vi "SetDisplayState.vi"(8 "Error In":errorcluster, 10 "Enabled?":bool, 11 "Keithley 6485 In":refnum<visa-resource-name>) -> (0 "Error Out":errorcluster, 3 "Keithley 6485 Out":refnum<visa-resource-name>)   [LabVIEW 2012, in "Keithley-6485.lvlib"]
uses:
  Keithley-6485.lvlib
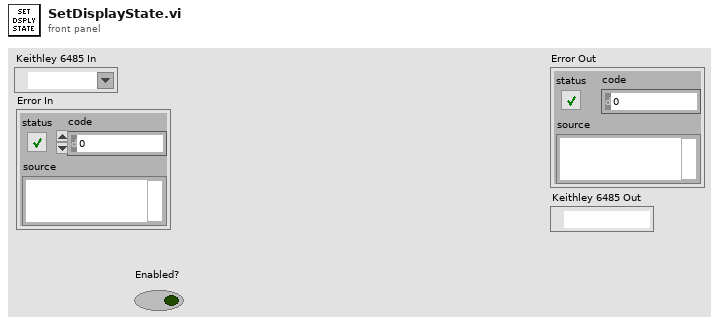
[diagram p1: front panel]
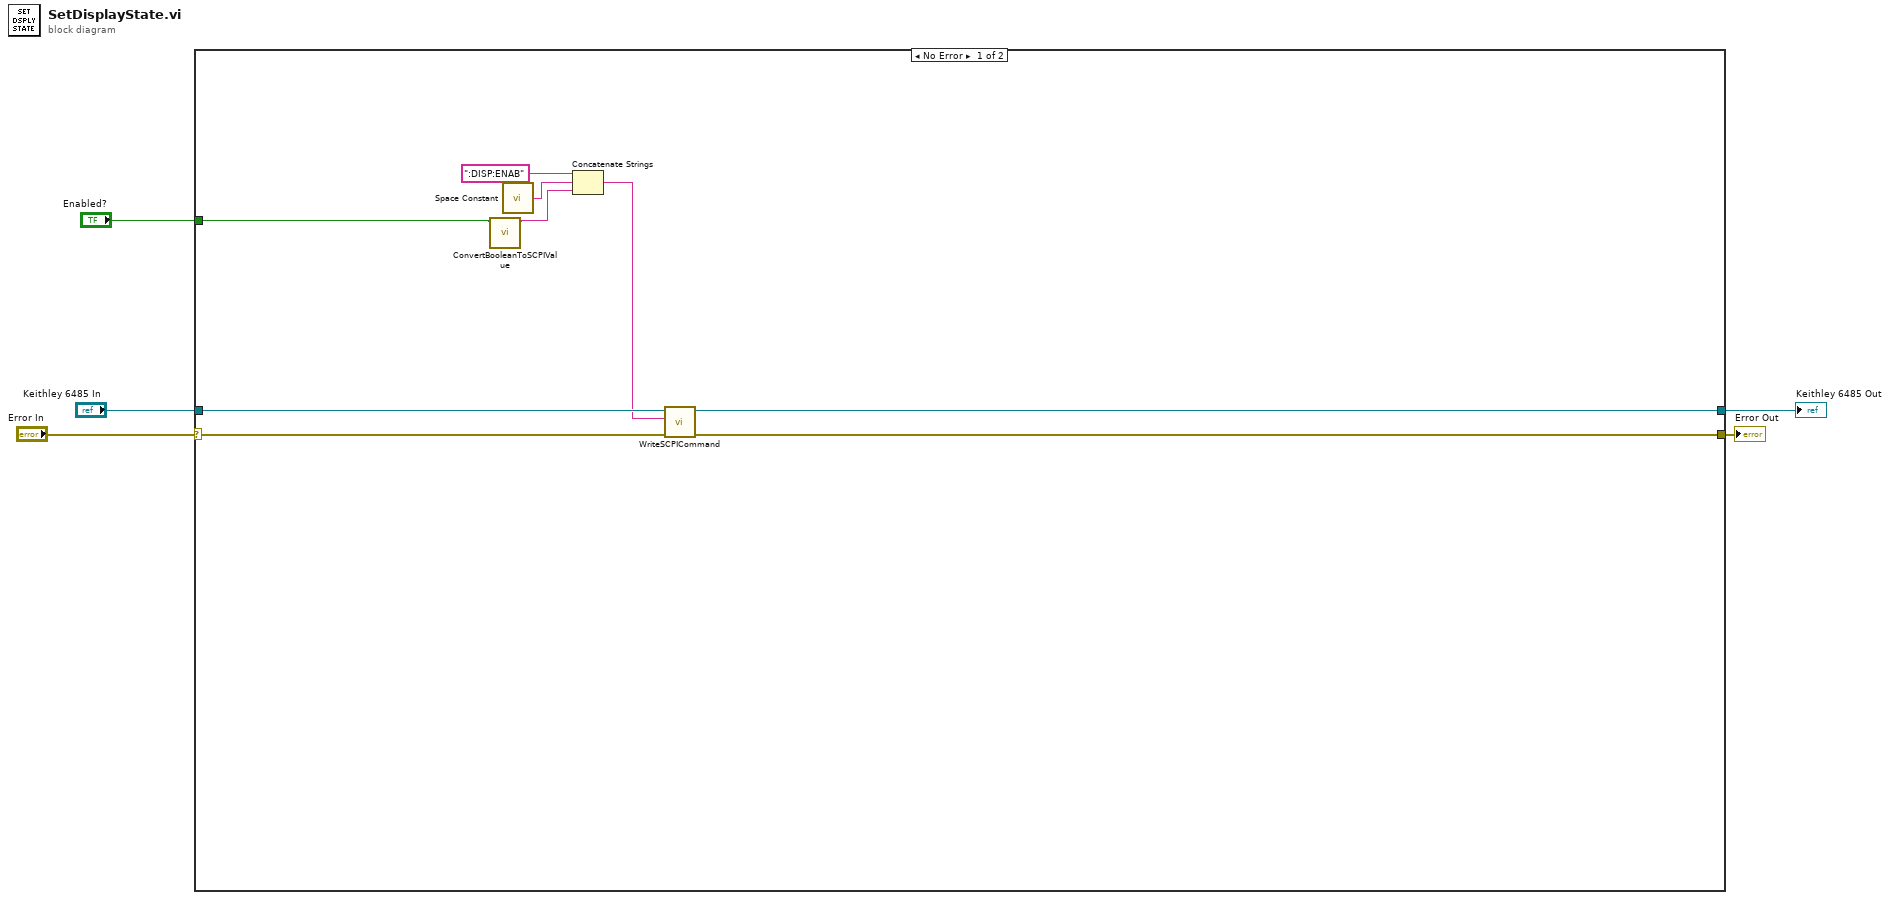
[diagram p0: block diagram]
diagram:
  n1 = case shown="No Error" "Error In" {
    selector: "Error In" -> [w9 w15]
    tunnel: "Keithley 6485 In" -> [w12 w16]
    tunnel: [w10 w15] -> w3
    tunnel: [w11 w16] -> w2
    tunnel: "Enabled?" -> [w6 _]
    frame No Error {
      n2 = call "ConvertBooleanToSCPIValue.vi"("Boolean"=w6) -> ("SCPI Value"=w7:string)  [unwired: 10 in]
      n3 = call <vilib>:"Space Constant.vi"() -> ("String"=w13:string)
      n4 = Concatenate Strings(":DISP:ENAB", w13, w7) -> (w8:string)
      n5 = call "WriteSCPICommand.vi"("Error In"=w9, "SCPI Command"=w8, "Keithley 6482 In"=w12) -> ("Error Out"=w10:errorcluster, "Keithley 6482 Out"=w11:refnum<visa-resource-name>)  [unwired: 7 in]
    }
    frame Error {
    }
  }
  "Error Out" <- w3
  "Keithley 6485 Out" <- w2
